vi "ActionVIOnPaste.vi"(6 "All Ptrs":T1[](array[typedef]) format="%.0x", 8 "error in (no error)":errorcluster, 10 "Parent":T1 format="%.0x", 11 "Ptr in":T1 format="%.0x") -> (0 "error out":errorcluster, 3 "Ptr out":T1 format="%.0x")   [LabVIEW 2024, in "Diagnostics Addon System Explorer.lvlib"]
uses:
  Diagnostics Addon System Explorer.lvlib
  <vilib>/NI VeriStand/Custom Device API/Custom Device Item Ref.ctl
  Types/FG.Action.ctl
  Addon Shared/SubVIs/Constants.vi
  <vilib>/NI VeriStand/Custom Device API/NI VeriStand - Get Item Parent.vi
  <vilib>/NI/NI VeriStand Advanced SysDef API/SysDef API/SysDef.Property.Set.vi
  <vilib>/NI/NI VeriStand Advanced SysDef API/_SubVIs/SysDef.Property.Set.U32.vi
  <vilib>/NI VeriStand/Custom Device API/NI VeriStand - Get Item Property.vi
  <vilib>/NI VeriStand/Custom Device API/Get Item Property (U32).vi
  <vilib>/NI VeriStand/Custom Device API/Custom Device API.lvlib
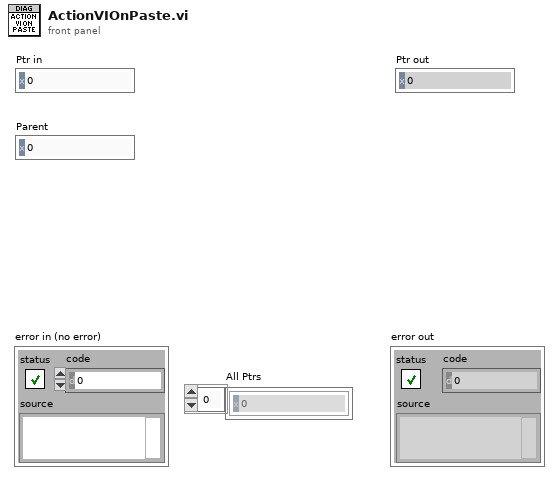
[diagram p1: front panel]
types:
  T1 = typedef "Custom Device API.lvlib/Custom Device Item Ref.ctl" = u64
  T2 = typedef "Diagnostics Addon System Explorer.lvlib/FG.Action.ctl" = enum16{"Get", "Set"}
  T3 = typedef "Diagnostics Addon Shared.lvlib/Type.ctl" = enum16{"DID", "CDID", "PID", "CPID", "Read Memory", "Write Memory", "IO Control", "Routine Start", "Routine Request", "Routine Stop", "User Defined", "DTC Control", "Clear DTCs", "Read DTCs", "Start DTCs", "DTC Change Count", "Tester Present", "Unlock ECU", "Reset ECU", "Diag Session Control", "Communication Control", "DPID Control", "Poll Control", "Diag Comm Port Control"}
  T4 = typedef "Custom Device API.lvlib/Custom Device Item Info.ctl" = cluster{"Name":string, "Is Channel":bool, "GUID":string, "Is Waveform":bool}
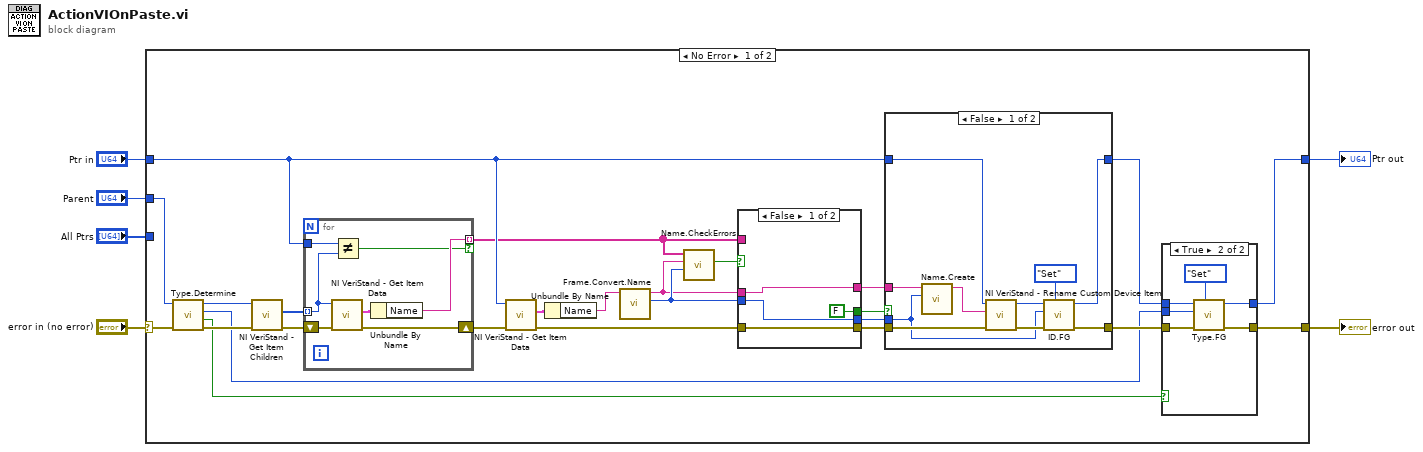
[diagram p0: block diagram]
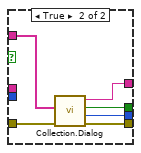
[diagram p2: hidden frame]
diagram:
  n1 = case shown="No Error" "error in (no error)" {
    selector: "error in (no error)" -> [w25 w70]
    tunnel: [w20 w70] -> w5
    tunnel: "Ptr in" -> [w12 w69]
    tunnel: [w16 w69] -> w3
    tunnel: "All Ptrs" -> [_ _]
    tunnel: "Parent" -> [w23 _]
    frame No Error {
      n2 = call "Type.Determine.vi"("error in (no error)"=w25, "Node Ptr"=w23) -> ("error out"=w24:errorcluster, "Found?"=w18:bool, "Type"=w19:T3, "Item Ref out"=w22:T1)  [unwired: 6 in]
      n3 = call <vilib>:"NI VeriStand - Get Item Children.vi"("error in (no error)"=w24, "Item Ref in"=w22) -> ("error out"=w31:errorcluster, "Child Refs"=w30:T1[])  [unwired: 6 in, 2 out]
      n4 = for {
        tunnel: [w66] -> w11 mode=indexing if=w62
        shift-right: [w65] -> w14
        shift-left: w31 -> [w67]
        tunnel: w30 -> [w63] mode=indexing
        tunnel: w12 -> [w64]
        n5 = call <vilib>:"NI VeriStand - Get Item Data.vi"("error in (no error)"=w67, "Item Ref in"=w63) -> ("error out"=w65:errorcluster, "Item Info"=w68:T4)  [unwired: 8 out]
        n6 = Not Equal?(x=w64, y=w63) -> (x != y?=w62:bool)
        n7 = Unbundle By Name(w68) -> ("Name"=w66:string)
      }
      n8 = call <vilib>:"NI VeriStand - Get Item Data.vi"("error in (no error)"=w14, "Item Ref in"=w12) -> ("error out"=w13:errorcluster, "Item Info"=w15:T4)  [unwired: 8 out]
      n9 = Unbundle By Name(w15) -> ("Name"=w10:string)
      n10 = call "Frame.Convert.Name.vi"("VS Frame Name"=w10) -> ("ID"=w8:u16, "Frame Name"=w7:string)  [unwired: 9 in]
      n11 = call "Name.CheckErrors.vi"("ID"=w8, "Name"=w7, "Existing Frames"=w11) -> ("Error?"=w9:bool)  [unwired: 7 in, 1 out]
      n12 = case shown="False" w9 {
        tunnel: [w33 w41] -> w29
        tunnel: [w34 w40] -> w28
        tunnel: [w35 w39] -> w27
        tunnel: [FALSE ("Cancel PID?") w38] -> w26
        tunnel: w13 -> [w33 w37]
        tunnel: w11 -> [_ w36]
        tunnel: w8 -> [w35 _]
        tunnel: w7 -> [w34 _]
        frame False {
        }
        frame True {
          n13 = call "Collection.Dialog.vi"("error in (no error)"=w37, "Existing PIDs"=w36) -> ("error out"=w41:errorcluster, "ID out"=w39:u16, "Cancel PID?"=w38:bool, "Name out"=w40:string)  [unwired: 6 in]
        }
      }
      n14 = case shown="False" w26 {
        tunnel: w12 -> [w58 w61]
        tunnel: [w52 w61] -> w17
        tunnel: [w54 w60] -> w21
        tunnel: w29 -> [w57 w60]
        tunnel: w28 -> [w56 _]
        tunnel: w27 -> [w50 _]
        frame False {
          n15 = call "Name.Create.vi"("PID Number"=w50, "PID Name"=w56) -> ("VS Name"=w59:string)  [unwired: 9 in]
          n16 = call <vilib>:"NI VeriStand - Rename Custom Device Item.vi"("error in (no error)"=w57, "New Name"=w59, "Item Ref in"=w58) -> ("error out"=w55:errorcluster, "Item Ref out"=w53:T1)  [unwired: 1 in, 6 out]
          n17 = call "ID.FG.vi"("Action"=FG.Action."Set", "error in (no error)"=w55, "ID"=w50, "Device Item Ref in"=w53) -> ("error out"=w54:errorcluster, "Device Item Ref out"=w52:T1)  [unwired: 5 in, 1 out]
        }
        frame True {
        }
      }
      n18 = case shown="True" w18 {
        tunnel: w21 -> [w42 w49]
        tunnel: [w42 w48] -> w20
        tunnel: w17 -> [w43 w47]
        tunnel: [w43 w46] -> w16
        tunnel: w19 -> [_ w44]
        frame False {
        }
        frame True {
          n19 = call "Type.FG.vi"("Action"=FG.Action."Set", "error in (no error)"=w49, "Type"=w44, "Device Item Ref in"=w47) -> ("error out"=w48:errorcluster, "Device Item Ref out"=w46:T1)  [unwired: 5 in, 1 out]
        }
      }
    }
    frame Error {
    }
  }
  "error out" <- w5
  "Ptr out" <- w3
